vi "Dynamic Set.vi"(6 "target resistance (ohm)":dbl=6000.0 format="%#_6p", 8 "error in (no error)":errorcluster, 9 "SET outfile":path=path "C:/Temp/SET_out.tmp", 10 "addr":i32, 11 "instrument handle":refnum<k15>) -> (0 "error out":errorcluster, 1 "final current (A)":dbl, 2 "final resistance (ohm)":dbl format="%#_6p", 3 "instrument handle out":refnum<k15>, 4 "SET?":bool, 5 "WL voltage (V)":dbl, 7 "BL voltage (V)":dbl)   [LabVIEW 2018]
uses:
  <instrlib>/niDigital/niDigital.llb/niDigital Burst Pattern (Burst Only).vi
  <vilib>/Utility/file.llb/Write Delimited Spreadsheet (DBL).vi
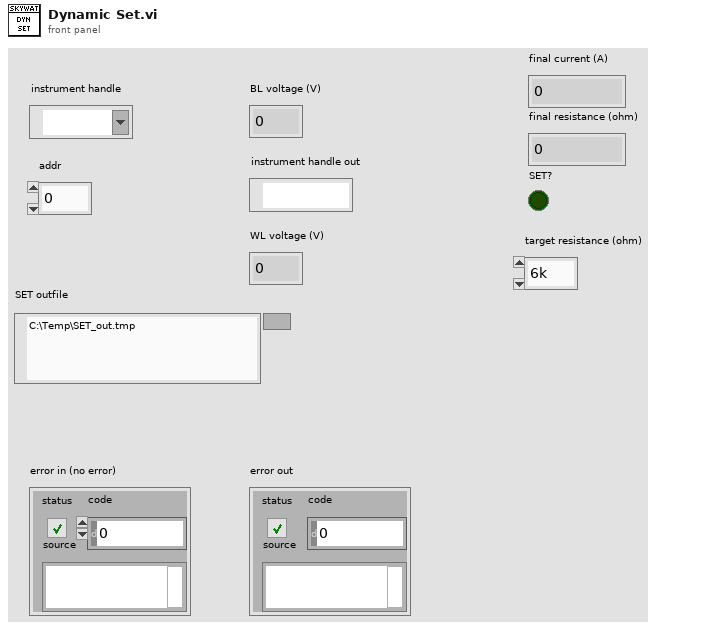
[diagram p1: front panel]
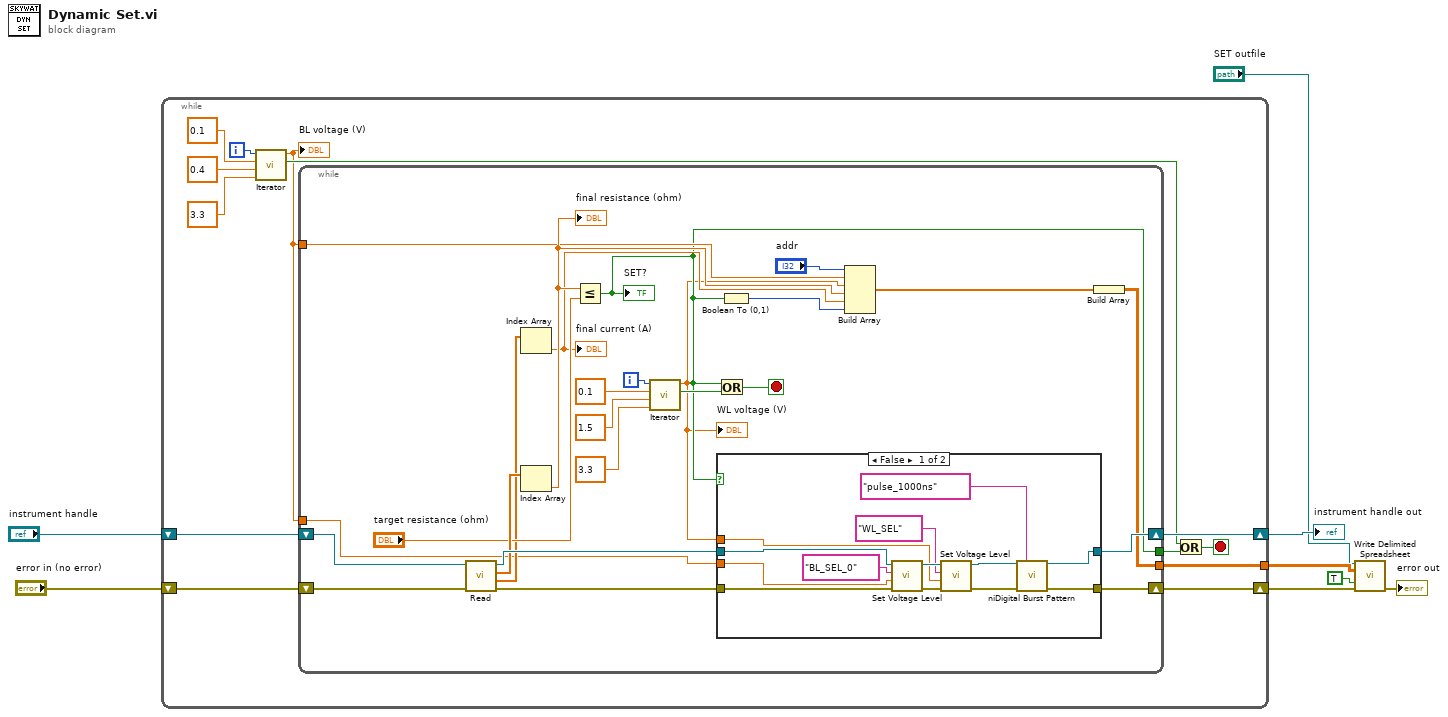
[diagram p0: block diagram]
diagram:
  n1 = while {
    shift-right: [w17] -> w6
    shift-left: "instrument handle" -> [w14]
    shift-right: [w16] -> w1
    shift-left: "error in (no error)" -> [w13]
    tunnel: [w9] -> w5
    i -> [w18]
    stop <- w19 stop-if-true
    n2 = call "Iterator.vi"("Final Value"=3.3 ("y"), "Initial Value"=0.4 ("y"), "Step"=0.1 ("x"), "i"=w18) -> ("End Loop"=w15:bool, "Current Value"=w10:dbl)  [unwired: 6 in]
    "BL voltage (V)" <- w10
    n3 = while {
      shift-right: [w45] -> w17
      shift-left: w14 -> [w41]
      shift-right: [w22] -> w16
      shift-left: w13 -> [w44]
      tunnel: w10 -> [w27]
      tunnel: [w26] -> w11
      tunnel: w10 -> [w24]
      tunnel: [w23] -> w9
      i -> [w40]
      stop <- w46 stop-if-true
      n4 = call "Read.vi"("error in (no error)"=w44, "instrument handle"=w41) -> ("error out"=w43:errorcluster, "currents (A)"=w33:dbl[], "resistances (ohm)"=w35:dbl[], "instrument handle out"=w42:refnum<k15>)  [unwired: 6 in]
      n5 = Index Array(array=w33) -> (element=w28:dbl)  [unwired: 1 in]
      "final current (A)" <- w28
      n6 = Index Array(array=w35) -> (element=w29:dbl)  [unwired: 1 in]
      "final resistance (ohm)" <- w29
      n7 = Less Or Equal?(x=w29, y="target resistance (ohm)") -> (x <= y?=w26:bool)
      "SET?" <- w26
      n8 = call "Iterator.vi"("Final Value"=3.3 ("y"), "Initial Value"=1.5 ("y"), "Step"=0.1 ("x"), "i"=w40) -> ("End Loop"=w36:bool, "Current Value"=w25:dbl)  [unwired: 6 in]
      "WL voltage (V)" <- w25
      n9 = Or(x=w26, y=w36) -> (x .or. y?=w46:bool)
      n10 = case shown="False" w26 {
        tunnel: [w59 w60] -> w22
        tunnel: [w58 w61] -> w45
        tunnel: w43 -> [w55 w60]
        tunnel: w42 -> [w54 w61]
        tunnel: w25 -> [w50 _]
        tunnel: w24 -> [w49 _]
        frame False {
          n11 = call "Set Voltage Level.vi"("error in (no error)"=w55, "level (V)"=w49, "channel list"="BL_SEL_0", "instrument handle"=w54) -> ("error out"=w57:errorcluster, "instrument handle out"=w56:refnum<k15>)  [unwired: 6 in]
          n12 = call "Set Voltage Level.vi"("error in (no error)"=w57, "level (V)"=w50, "channel list"="WL_SEL", "instrument handle"=w56) -> ("error out"=w47:errorcluster, "instrument handle out"=w48:refnum<k15>)  [unwired: 6 in]
          n13 = call-poly <instrlib>:"niDigital Burst Pattern.vi"("instrument handle"=w48, "start label"="pulse_1000ns", "error in"=w47) -> ("instrument handle out"=w58:refnum<k15>, "error out"=w59:errorcluster)  [unwired: 11 in]
        }
        frame True {
        }
      }
      n14 = Boolean To (0,1)(Boolean=w26) -> (0, 1=w32:i16)
      n15 = Build Array("addr", w27, w25, w29, w28, w32) -> (w31:dbl[])
      n16 = Build Array(w31) -> (w23:dbl[][])
    }
    n17 = Or(x=w15, y=w11) -> (x .or. y?=w19:bool)
  }
  "instrument handle out" <- w6
  n18 = call-poly <vilib>:"Write Delimited Spreadsheet.vi"("file path (dialog if empty)"="SET outfile", "2D data"=w5, "append to file? (new file:F)"=TRUE, "error in (no error)"=w1) -> ("error out"=→"error out":errorcluster)  [unwired: 10 in, 1 out]
